vi "CAT Panel - MSR.vi"() -> ()   [LabVIEW 2012]
uses:
  <vilib>/Platform/TimedLoop/XDataNode/wakeup.ctl
  <vilib>/Platform/TimedLoop/XDataNode/XDNodeRunTimeDep.lvlib
  <vilib>/Platform/TimedLoop/XDataNode/nitl_modes.ctl
  <vilib>/Platform/TimedLoop/XDataNode/timing_clust.ctl
  <vilib>/Platform/TimedLoop/XDataNode/XDataNode.xnode
  Type Defs/Data Reading.ctl
  Type Defs/4 Way Button.ctl
  Output Timer/Output Timer.lvclass
  Type Defs/Alt Digit 100 New.ctl
  Type Defs/Alt Control.ctl
  Type Defs/All Timers.ctl
  Type Defs/Final Output for Dispaly.ctl
  Type Defs/Alt Display Large.ctl
  Type Defs/Final Output.ctl
  Type Defs/Output Values.ctl
  Type Defs/Output Switches.ctl
  Type Defs/CO2 Settings.ctl
  Type Defs/AD Settings.ctl
  Type Defs/Mode Select.ctl
  Type Defs/Action Time.ctl
  Type Defs/Timer Control.ctl
  Type Defs/Current Alt Set.ctl
  Altitude/Altitude.xctl
  Mode Control/Mode.xctl
panel:
  out "read string":string="Ver. 0.1, Feb 10 2013, 23:27:07\r\n"
  in  "Tab Control":T1(tab)=enum."CO2 Settings"
  in  "Other Outputs":cluster{"Alarm":bool, "Heater":bool}
  out "CO2 ppm":u32(slide)=831 scale=0.0..10000.0
  out "Alt Dif M":dbl(slide)=1598.2180776729308 scale=-1000.0..1000.0 scale format="%.1f"
  out "AD Output":T2
  out "AD State":T2
  out "Data Read":T3={"Date"="03/29/13", "Time"="15:49:08", "CO2- ppm"=831, "Last Ctrl Word"=4194304, "O2-1 ppm"=209373, "O2-2 ppm"=209370, "Temp MB"=21.72, "Temp Sensor Module"=23.23, "Press mB"=835.6} {"Last Ctrl Word" format="%.0x"}
  out "Force Output":T2
  out "Final Output":T2
  out "Force State":T2
  in  "CO2 Settings":T4={"Run C1"={"A-1,  1"=inf, "A-3,  2"=inf, "A-4, 3"=9000.0, "A-5, 4"=8800.0, "ABCD-7, 5"=9600.0, "A-8, 6"=9200.0, "B-1,  7"=3400.0, "B-3, 8"=3400.0, "B-4,  9"=9000.0, "B-5, 10"=8800.0, "B-8, 11"=9200.0, "C-1, 12"=1800.0, "C-3, 13"=1800.0, "C-4, 14"=9000.0, "C-5,  15"=8800.0, "C-8, 16"=9200.0, "D-1, 17"=inf, "D-3, 18"=3400.0, "D-4,  19"=1800.0, "D-5,  20"=7000.0, "D-8,  21"=9200.0}, "Run C2"={"A-1,  1"=inf, "A-3,  2"=inf, "A-4, 3"=8800.0, "A-5, 4"=8600.0, "ABCD-7, 5"=9400.0, "A-8, 6"=9000.0, "B-1,  7"=3000.0, "B-3, 8"=3000.0, "B-4,  9"=8800.0, "B-5, 10"=8600.0, "B-8, 11"=9000.0, "C-1, 12"=1400.0, "C-3, 13"=1400.0, "C-4, 14"=8800.0, "C-5,  15"=8600.0, "C-8, 16"=9000.0, "D-1, 17"=inf, "D-3, 18"=3000.0, "D-4,  19"=1400.0, "D-5,  20"=6600.0, "D-8,  21"=9000.0}, "Hold C3"={"A-1,  1"=1800.0, "A-3,  2"=1800.0, "A-4, 3"=9000.0, "A-5, 4"=8800.0, "ABCD-7, 5"=9600.0, "A-8, 6"=9200.0, "B-1,  7"=3400.0, "B-3, 8"=3400.0, "B-4,  9"=9000.0, "B-5, 10"=8800.0, "B-8, 11"=9200.0, "C-1, 12"=1800.0, "C-3, 13"=1800.0, "C-4, 14"=9000.0, "C-5,  15"=8800.0, "C-8, 16"=9200.0, "D-1, 17"=1800.0, "D-3, 18"=3400.0, "D-4,  19"=1800.0, "D-5,  20"=7000.0, "D-8,  21"=9200.0}, "Hold C4"={"A-1,  1"=1400.0, "A-3,  2"=1400.0, "A-4, 3"=8800.0, "A-5, 4"=8600.0, "ABCD-7, 5"=9400.0, "A-8, 6"=9000.0, "B-1,  7"=3000.0, "B-3, 8"=3000.0, "B-4,  9"=8800.0, "B-5, 10"=8600.0, "B-8, 11"=9000.0, "C-1, 12"=1400.0, "C-3, 13"=1400.0, "C-4, 14"=8800.0, "C-5,  15"=8600.0, "C-8, 16"=9000.0, "D-1, 17"=1400.0, "D-3, 18"=3000.0, "D-4,  19"=1400.0, "D-5,  20"=6600.0, "D-8,  21"=9000.0}, "High CO2 Forces "={"A-1, 1"=TRUE, "A-3, 2"=TRUE, "A-4, 3"=FALSE, "A-5, 4"=TRUE, "ABCD-7, 5"=FALSE, "A-8, 6"=TRUE, "B-1,  7"=TRUE, "B-3, 8"=TRUE, "B-4, 9"=FALSE, "B-5, 10"=TRUE, "B-8,  11"=TRUE, "C-1, 12"=TRUE, "C-3, 13"=TRUE, "C-4,  14"=FALSE, "C-5,  15"=TRUE, "C-8, 16"=TRUE, "D-1, 17"=TRUE, "D-3, 18"=TRUE, "D-4, 19"=TRUE, "D-5,  20"=TRUE, "D-8,  21"=TRUE}}
  in  "AD Settings":T7={"Set Point Force"={"A-1,  1"=inf, "A-3,  2"=inf, "A-4, 3"=inf, "A-5, 4"=inf, "ABCD-7, 5"=inf, "A-8, 6"=inf, "B-1,  7"=inf, "B-3, 8"=inf, "B-4,  9"=inf, "B-5, 10"=inf, "B-8, 11"=inf, "C-1, 12"=inf, "C-3, 13"=inf, "C-4, 14"=inf, "C-5,  15"=inf, "C-8, 16"=inf, "D-1, 17"=inf, "D-3, 18"=inf, "D-4,  19"=inf, "D-5,  20"=6000.0, "D-8,  21"=inf}, "Run A1"={"A-1,  1"=inf, "A-3,  2"=inf, "A-4, 3"=50.0, "A-5, 4"=inf, "ABCD-7, 5"=150.0, "A-8, 6"=60.0, "B-1,  7"=0.0, "B-3, 8"=0.0, "B-4,  9"=50.0, "B-5, 10"=inf, "B-8, 11"=60.0, "C-1, 12"=15.0, "C-3, 13"=15.0, "C-4, 14"=50.0, "C-5,  15"=inf, "C-8, 16"=60.0, "D-1, 17"=inf, "D-3, 18"=0.0, "D-4,  19"=15.0, "D-5,  20"=0.0, "D-8,  21"=700.0}, "Run A2"={"A-1,  1"=inf, "A-3,  2"=inf, "A-4, 3"=-30.0, "A-5, 4"=inf, "ABCD-7, 5"=80.0, "A-8, 6"=15.0, "B-1,  7"=-80.0, "B-3, 8"=-80.0, "B-4,  9"=-30.0, "B-5, 10"=inf, "B-8, 11"=15.0, "C-1, 12"=-50.0, "C-3, 13"=-50.0, "C-4, 14"=-30.0, "C-5,  15"=inf, "C-8, 16"=15.0, "D-1, 17"=inf, "D-3, 18"=0.0, "D-4,  19"=-50.0, "D-5,  20"=-80.0, "D-8,  21"=650.0}, "Hold A3"={"A-1,  1"=0.0, "A-3,  2"=0.0, "A-4, 3"=50.0, "A-5, 4"=inf, "ABCD-7, 5"=150.0, "A-8, 6"=60.0, "B-1,  7"=-150.0, "B-3, 8"=-150.0, "B-4,  9"=50.0, "B-5, 10"=inf, "B-8, 11"=60.0, "C-1, 12"=-200.0, "C-3, 13"=-200.0, "C-4, 14"=50.0, "C-5,  15"=inf, "C-8, 16"=60.0, "D-1, 17"=0.0, "D-3, 18"=-150.0, "D-4,  19"=-200.0, "D-5,  20"=-200.0, "D-8,  21"=650.0}, "Hold A4"={"A-1,  1"=-150.0, "A-3,  2"=-150.0, "A-4, 3"=-30.0, "A-5, 4"=inf, "ABCD-7, 5"=80.0, "A-8, 6"=15.0, "B-1,  7"=-250.0, "B-3, 8"=-250.0, "B-4,  9"=-30.0, "B-5, 10"=inf, "B-8, 11"=15.0, "C-1, 12"=-300.0, "C-3, 13"=-300.0, "C-4, 14"=-30.0, "C-5,  15"=inf, "C-8, 16"=15.0, "D-1, 17"=-150.0, "D-3, 18"=-250.0, "D-4,  19"=-300.0, "D-5,  20"=-300.0, "D-8,  21"=650.0}, "High AD Diff "={"A-1, 1"=FALSE, "A-3, 2"=FALSE, "A-4, 3"=FALSE, "A-5, 4"=TRUE, "ABCD-7, 5"=FALSE, "A-8, 6"=TRUE, "B-1,  7"=FALSE, "B-3, 8"=FALSE, "B-4, 9"=FALSE, "B-5, 10"=TRUE, "B-8,  11"=TRUE, "C-1, 12"=FALSE, "C-3, 13"=FALSE, "C-4,  14"=FALSE, "C-5,  15"=TRUE, "C-8, 16"=TRUE, "D-1, 17"=FALSE, "D-3, 18"=FALSE, "D-4, 19"=FALSE, "D-5,  20"=FALSE, "D-8,  21"=TRUE}, "Delay S"={"A-1,  1"=30.0, "A-3,  2"=30.0, "A-4, 3"=1.0, "A-5, 4"=1.0, "ABCD-7, 5"=1.0, "A-8, 6"=1.0, "B-1,  7"=30.0, "B-3, 8"=30.0, "B-4,  9"=1.0, "B-5, 10"=1.0, "B-8, 11"=1.0, "C-1, 12"=30.0, "C-3, 13"=30.0, "C-4, 14"=1.0, "C-5,  15"=1.0, "C-8, 16"=1.0, "D-1, 17"=30.0, "D-3, 18"=30.0, "D-4,  19"=30.0, "D-5,  20"=30.0, "D-8,  21"=1.0}}
  in  "Main States":T8(tab)=enum."Setup"
  out "ALT DISPLAY":sgl format="%#.0f"
  out "CURRENT ALT SET":T9=1598 format="%#.0f"
  in  "Mode 1":T10
  in  "Confirm Now 2":bool
  out "Carbon Dioxide  %":sgl=0.0831 format="%.3f"
  in  "ALT SET 2":T11 {"Alt Digit 100" min=0 max=9 step=1; "Alt Digit 100" min=0 max=9 step=1; "Alt Digit 100" min=0 max=9 step=1; "Alt Digit 100" min=0 max=9 step=1; "Alt Digit 100" min=0 max=9 step=1}
  out "ALT DISPLAY 2":T13=1598.218 format="%#.0f"
  out "CURRENT ALT SET 2":T9=1598 format="%#.0f"
  in  "Mode":T10
  out "Time":string="15:49:02"
  in  "Add Note":bool
  out "Final Output Display":T14
  out "CO2 Chart":dbl(graph)=0.0831
  out "Temp C":sgl=21.69
  out "Press mB":sgl=835.53
  out "Date":string="03/29/13"
  out "Alt Chart":dbl(graph)=1598.2180776729308
  out "Carbon Dioxide":sgl=0.0831 format="%.3g"
  in  "Confirm Now":bool
  in  "Notes":string
  in  "ALT SET":T11 {"Alt Digit 100" min=0 max=9 step=1; "Alt Digit 100" min=0 max=9 step=1; "Alt Digit 100" min=0 max=9 step=1; "Alt Digit 100" min=0 max=9 step=1; "Alt Digit 100" min=0 max=9 step=1}
  out "Altitude":sgl=1598.218 format="%#.0f"
  out "O2%":dbl=21.4333 format="%.1f"
  in  "Timers":T15 {"Timer 4"."Action Time" format="%<%H:%M>t"; "Timer 3"."Action Time" format="%<%H:%M>t"; "Timer 2"."Action Time" format="%<%H:%M>t"; "Timer"."Action Time" format="%<%H:%M>t"}
  in  "Datalog File":path
  in  "Period mS":i64=6000
  in  "Stop Button":bool
  in  "West ON/Std OFF":bool
  out "error out":errorcluster
  out "Cycles":i32=5
  in  "Mode Select":T18
  in  "Set Point Alt":sgl min=0 max=10000 step=1
  # "CAT 100.8"
  # "Current Effective Altitude in  Meters"
  # "M\nE\nT\nE\nR\nS"
  # "%"
  # "Channel A"
  # "Channel B"
  # "Channel C"
  # "Channel D"
  # "1"
  # "1"
  # "1"
  # "1"
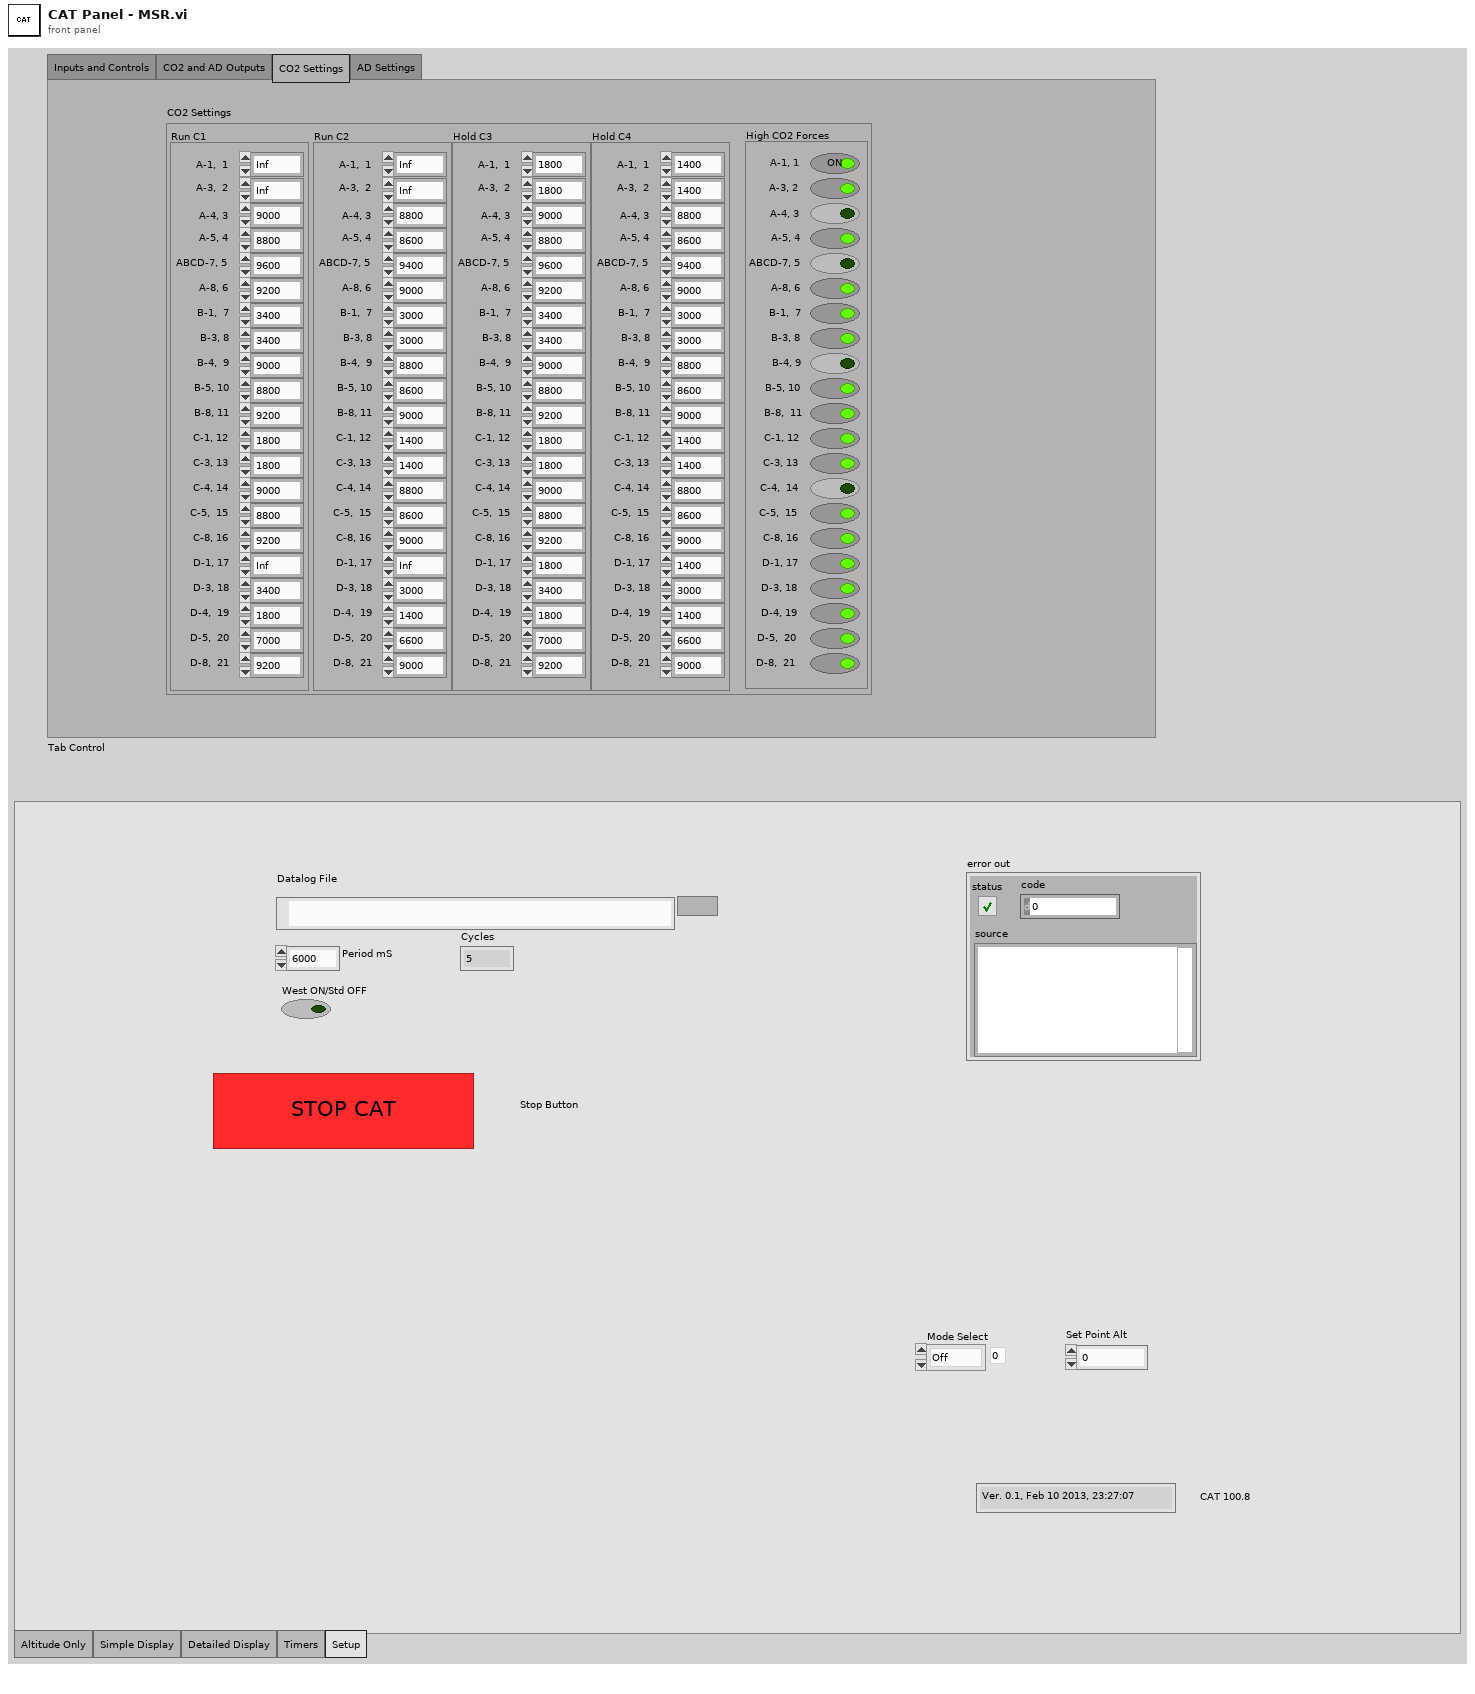
[diagram p1: front panel]
types:
  T1 = enum32{"Inputs and Controls", "CO2 and AD Outputs", "CO2 Settings", "AD Settings"}
  T2 = typedef "Final Output.ctl" = cluster{"Main 1":bool, "Main 2":bool, "Recirc  3":bool, "Scrub 4":bool, "O2 5":bool, "Vent 6":bool, "Boost A 7":bool, "Boost A 8":bool, "Recirc  9":bool, "Scrub 10":bool, "Vent 11":bool, "Boost B 12":bool, "Boost B 13":bool, "Recirc 14":bool, "Scrub 15":bool, "Vent 16":bool, "Main 17":bool, "Boost A 18":bool, "Boost B 19":bool, "Boost F 20":bool, "Vent 2 21":bool}
  T3 = typedef "Data Reading.ctl" = cluster{"Date":string, "Time":string, "CO2- ppm":u32, "Last Ctrl Word":u32, "O2-1 ppm":u32, "O2-2 ppm":u32, "Temp MB":sgl, "Temp Sensor Module":sgl, "Press mB":sgl}
  T4 = typedef "CO2 Settings.ctl" = cluster{"Run C1":T5, "Run C2":T5, "Hold C3":T5, "Hold C4":T5, "High CO2 Forces ":T6}
  T5 = typedef "Output Values.ctl" = cluster{"A-1,  1":dbl, "A-3,  2":dbl, "A-4, 3":dbl, "A-5, 4":dbl, "ABCD-7, 5":dbl, "A-8, 6":dbl, "B-1,  7":dbl, "B-3, 8":dbl, "B-4,  9":dbl, "B-5, 10":dbl, "B-8, 11":dbl, "C-1, 12":dbl, "C-3, 13":dbl, "C-4, 14":dbl, "C-5,  15":dbl, "C-8, 16":dbl, "D-1, 17":dbl, "D-3, 18":dbl, "D-4,  19":dbl, "D-5,  20":dbl, "D-8,  21":dbl}
  T6 = typedef "Output Switches.ctl" = cluster{"A-1, 1":bool, "A-3, 2":bool, "A-4, 3":bool, "A-5, 4":bool, "ABCD-7, 5":bool, "A-8, 6":bool, "B-1,  7":bool, "B-3, 8":bool, "B-4, 9":bool, "B-5, 10":bool, "B-8,  11":bool, "C-1, 12":bool, "C-3, 13":bool, "C-4,  14":bool, "C-5,  15":bool, "C-8, 16":bool, "D-1, 17":bool, "D-3, 18":bool, "D-4, 19":bool, "D-5,  20":bool, "D-8,  21":bool}
  T7 = typedef "AD Settings.ctl" = cluster{"Set Point Force":T5, "Run A1":T5, "Run A2":T5, "Hold A3":T5, "Hold A4":T5, "High AD Diff ":T6, "Delay S":T5}
  T8 = enum32{"Altitude Only", "Simple Display", "Detailed Display", "Timers", "Setup"}
  T9 = typedef "Current Alt Set.ctl" = i32
  T10 = typedef "4 Way Button.ctl" = cluster{"Off":bool, "Standby":bool, "Hold":bool, "Run":bool}
  T11 = typedef "Alt Control.ctl" = cluster{"Alt Digit 100":T12, "Alt Digit 100":T12, "Alt Digit 100":T12, "Alt Digit 100":T12, "Alt Digit 100":T12}
  T12 = typedef "Alt Digit 100 New.ctl" = i8
  T13 = typedef "Alt Display Large.ctl" = sgl
  T14 = typedef "Final Output for Dispaly.ctl" = cluster{"A-1,  1":bool, "A-3,  2":bool, "A-4, 3":bool, "A-5, 4":bool, "ABCD-7, 5":bool, "A-8, 6":bool, "B-1,  7":bool, "B-3, 8":bool, "B-4,  9":bool, "B-5, 10":bool, "B-8, 11":bool, "C-1, 12":bool, "C-3, 13":bool, "C-4, 14":bool, "C-5,  15":bool, "C-8, 16":bool, "A-1, 17":bool, "D-3, 18":bool, "D-4,  19":bool, "D-5,  20":bool, "D-8,  21":bool}
  T15 = typedef "All Timers.ctl" = cluster{"Timer":T16, "Timer 2":T16, "Timer 3":T16, "Timer 4":T16}
  T16 = typedef "Timer Control.ctl" = cluster{"Sun":bool, "Timer":bool, "Altitude":sgl, "Action Time":T17, "Mon":bool, "Tues":bool, "Wed":bool, "Thur":bool, "Fri":bool, "Sat":bool, "Mode":enum8{"Off", "Stby", "Hold", "Run"}}
  T17 = typedef "Action Time.ctl" = dbl
  T18 = typedef "Mode Select.ctl" = enum8{"Off", "Stby", "Hold", "Run"}
  T19 = cluster{"Main 1":bool, "Main 2":bool, "Recirc  3":bool, "Boost A 7":bool, "Recirc  9":bool, "Scrub 4":bool, "Scrub 10":bool, "O2 5":bool, "Vent 6":bool, "Boost A 8":bool, "Vent 11":bool, "Boost B 12":bool, "Boost B 13":bool, "Recirc 14":bool, "Scrub 15":bool, "Vent 16":bool, "Main 17":bool, "Boost A 18":bool, "Boost B 19":bool, "Boost F 20":bool, "Vent 2 21":bool}
  T20 = typedef "XDNodeRunTimeDep.lvlib/timing_clust.ctl" = cluster{"Expected End [f-1]":u64, "Actual End [f-1]":u64, "Finished Late? [f-1]":bool, "Expected End [i-1]":u64, "Actual End [i-1]":u64, "Finished Late? [i-1]":bool, "Expected Start [i]":u64, "Actual Start [i]":u64, "Expected Start [f]":u64, "Actual Start [f]":u64, "Source Name":string, "Structure Name":string, "Period":i64, "Deadline":i64, "Offset":i64, "Start":i64, "Priority":i32, "Timeout":i32, "Mode":T21, "Wakeup Reason":T22, "Error":errorcluster, "Source Type":string, "Secondary Source Type":string, "Global End Time":u64, "Global Start Time":u64, "Frame Duration":u64, "Iteration Duration":u64, "Assigned CPU":i32, "I/O Scan Engine Mode":u32}
  T21 = typedef "XDNodeRunTimeDep.lvlib/nitl_modes.ctl" = enum32{"No Change", "Process missed periods, maintain original phase", "Discard missed periods, maintain original phase", "Process missed periods, ignore original phase", "Discard missed periods, ignore original phase"}
  T22 = typedef "XDNodeRunTimeDep.lvlib/wakeup.ctl" = enum32{"Normal", "Aborted", "Asynchronous wakeup", "Timing source error", "Timed loop error", "Timeout"}
  T23 = cluster{"A-1,  1":bool, "A-3,  2":bool, "A-4, 3":bool, "A-5, 4":bool, "ABCD-7, 5":bool, "A-8, 6":bool, "B-1,  7":bool, "B-3, 8":bool, "B-4,  9":bool, "B-5, 10":bool, "B-8, 11":bool, "C-1, 12":bool, "C-3, 13":bool, "C-4, 14":bool, "C-5,  15":bool, "C-8, 16":bool, "D-1, 17":bool, "D-3, 18":bool, "D-4,  19":bool, "D-5,  20":bool, "D-8,  21":bool}
  T24 = cluster{bool, bool, bool, bool, bool, bool, bool, bool, bool, bool, bool, bool, bool, bool, bool, bool, bool, bool, bool, bool, bool}
  T25 = cluster{"[0]":bool, "[1]":bool, "[2]":bool, "[3]":bool, "[4]":bool, "[5]":bool, "[6]":bool, "[7]":bool, "[8]":bool, "[9]":bool, "[10]":bool, "[11]":bool, "[12]":bool, "[13]":bool, "[14]":bool, "[15]":bool, "[16]":bool, "[17]":bool, "[18]":bool, "[19]":bool, "[20]":bool}
  T26 = cluster{"Date":string, "Time":string, "CO2- ppm":u32, "Last Ctrl Word":u32, "O2-1 ppm":u32, "O2-2 ppm":u32, "Temp MB":sgl, "Temp Sensor Module":sgl, "Press mB":sgl}
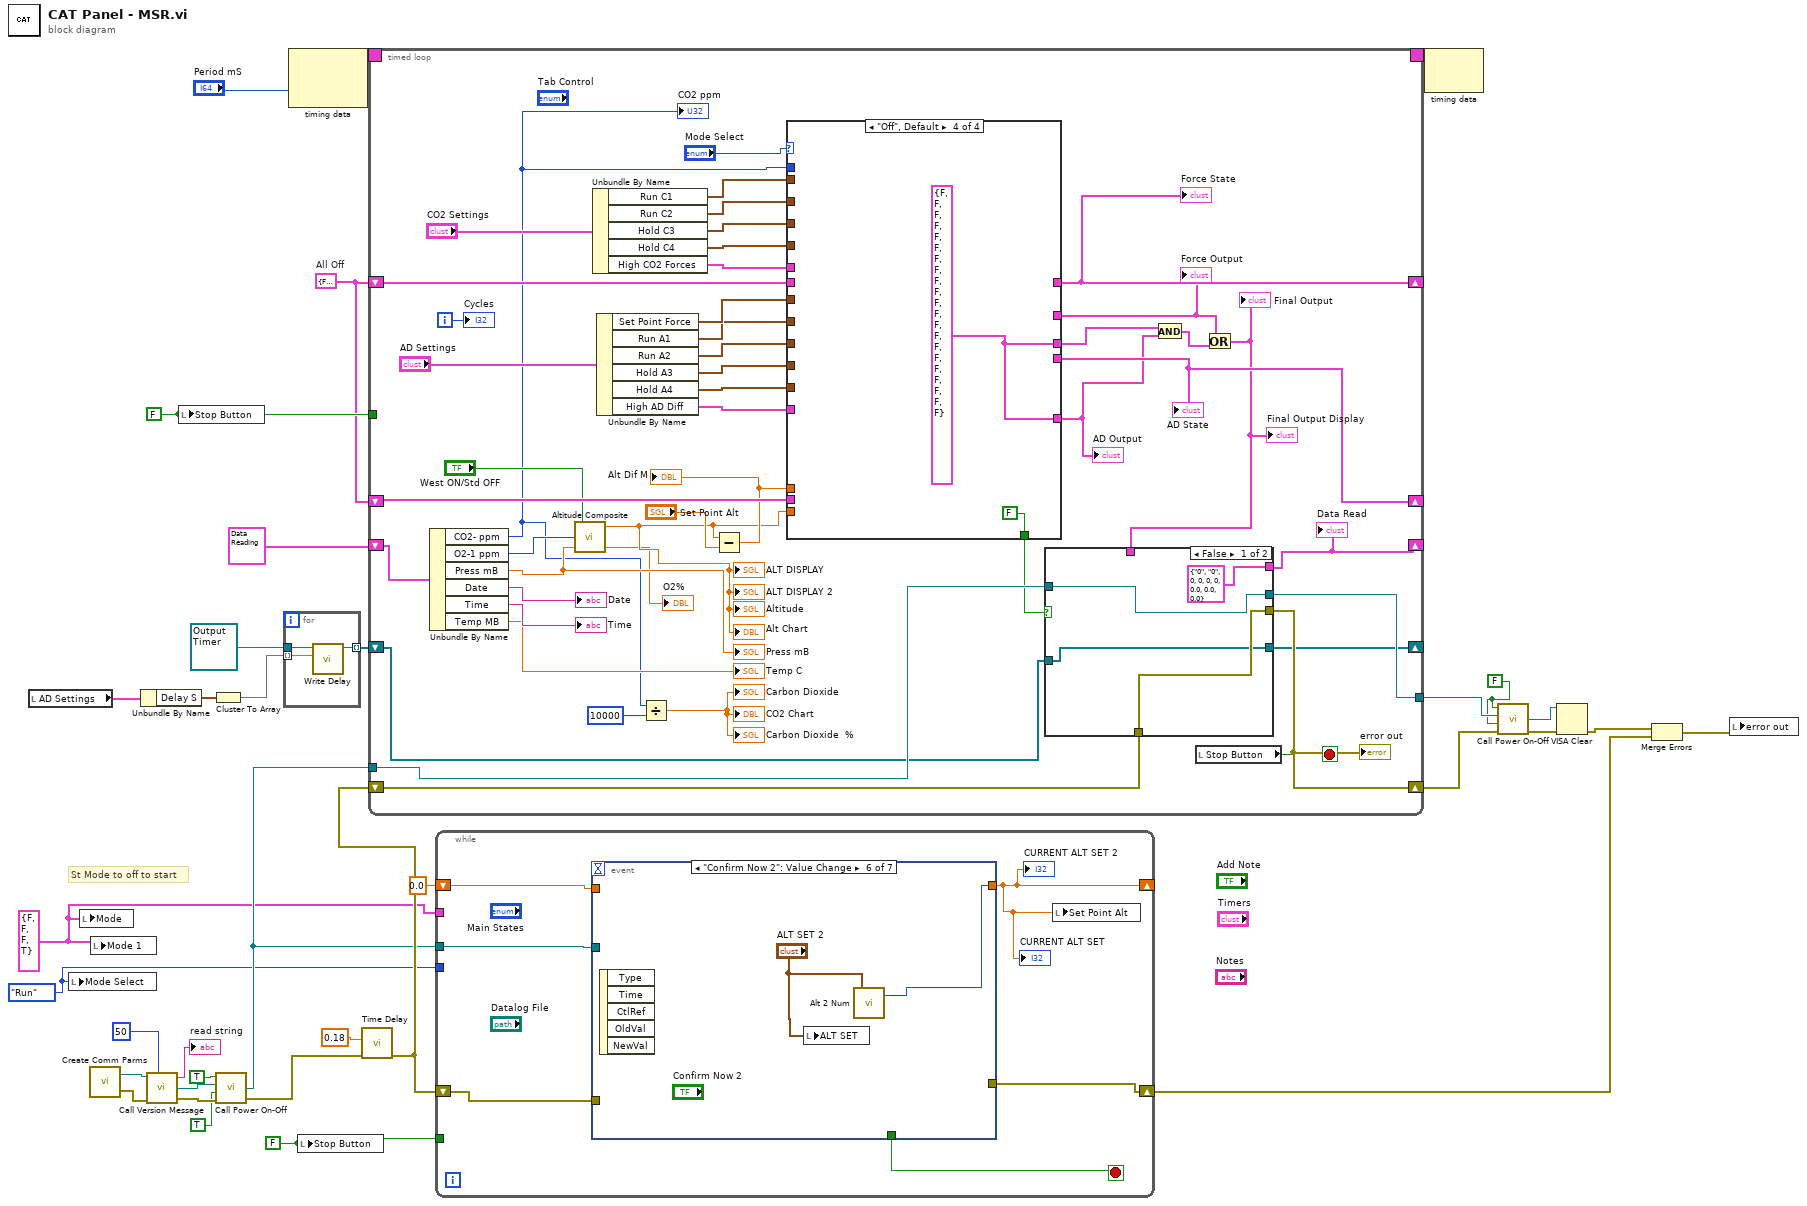
[diagram p0: block diagram]
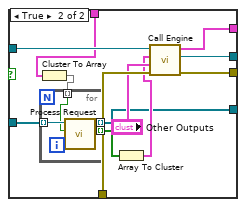
[diagram p2: hidden frame]
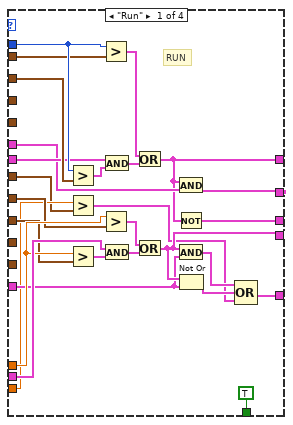
[diagram p3: hidden frame]
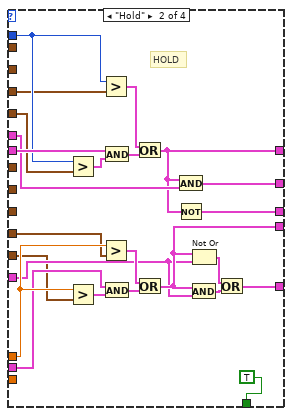
[diagram p4: hidden frame]
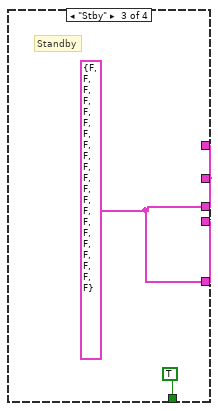
[diagram p5: hidden frame]
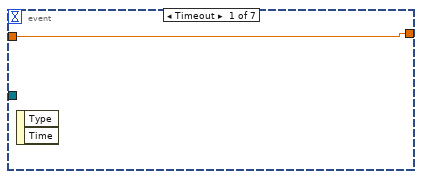
[diagram p6: hidden frame]
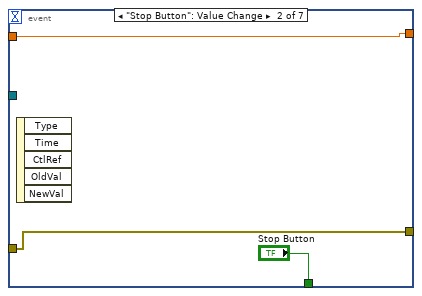
[diagram p7: hidden frame]
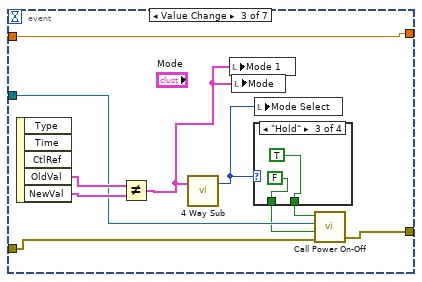
[diagram p8: hidden frame]
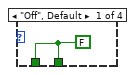
[diagram p9: hidden frame]
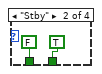
[diagram p10: hidden frame]
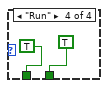
[diagram p11: hidden frame]
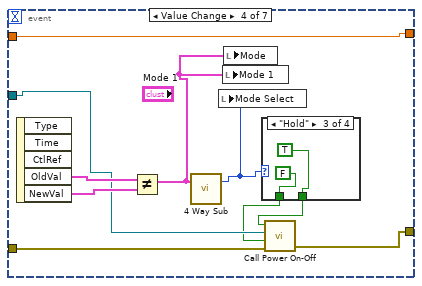
[diagram p12: hidden frame]
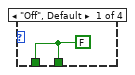
[diagram p13: hidden frame]
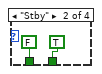
[diagram p14: hidden frame]
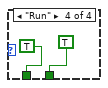
[diagram p15: hidden frame]
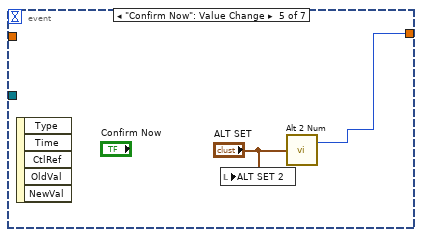
[diagram p16: hidden frame]
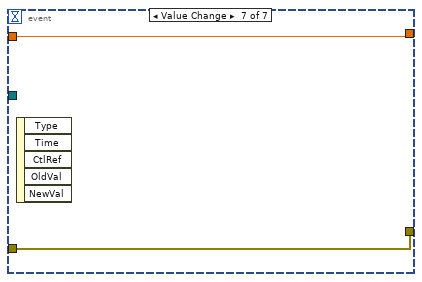
[diagram p17: hidden frame]
diagram:
  w1 = FALSE ("Leave CAT On/Off at Program Exit")
  w12 = T10 {"Off"=FALSE, "Standby"=FALSE, "Hold"=FALSE, "Run"=TRUE} ("Mode 1")
  w13 = enum8{"Off", "Stby", "Hold", "Run"}."Run" ("Mode Select")
  w31 = FALSE ("Stop Button")
  w32 = FALSE ("Stop Button")
  w30 = T19 {"Main 1"=FALSE, "Main 2"=FALSE, "Recirc  3"=FALSE, "Boost A 7"=FALSE, "Recirc  9"=FALSE, "Scrub 4"=FALSE, "Scrub 10"=FALSE, "O2 5"=FALSE, "Vent 6"=FALSE, "Boost A 8"=FALSE, "Vent 11"=FALSE, "Boost B 12"=FALSE, "Boost B 13"=FALSE, "Recirc 14"=FALSE, "Scrub 15"=FALSE, "Vent 16"=FALSE, "Main 17"=FALSE, "Boost A 18"=FALSE, "Boost B 19"=FALSE, "Boost F 20"=FALSE, "Vent 2 21"=FALSE}  # All Off
  # "St Mode to off to start"
  n1 = local read "AD Settings"() -> (w11:T7)
  n2 = local write "Mode Select"(w13) -> ()
  n3 = local write "Mode"(w12) -> ()
  n4 = call "Create Comm Parms.vi"() -> ("error out"=w19:errorcluster, "VISA resource name out"=w17:refnum<visa-resource-name>)  [unwired: 2 in]
  n5 = local write "Mode 1"(w12) -> ()
  n6 = Unbundle By Name(w11) -> ("Delay S"=w10:T5)
  n7 = call "Call Version Message.vi"("VISA resource name out"=w17, "delay before read (ms)"=u32 50, "error in"=w19) -> ("read string"=→"read string":string, "VISA resource name out 2"=w16:refnum<visa-resource-name>, "error out"=w18:errorcluster)  [unwired: 2 in, 1 out]
  n8 = local write "Stop Button"(w32) -> ()
  n9 = Cluster To Array(cluster=w10) -> (array=w9:dbl[])
  n10 = call "Call Power On-Off.vi"("error in"=w18, "Warmup if ON"=TRUE, "VISA resource name"=w16, "On/Off"=TRUE) -> ("error out"=w28:errorcluster, "VISA resource name out"=w22:refnum<visa-resource-name>)  [unwired: 1 in]
  n11 = for {
    tunnel: w9 -> [w37] mode=indexing
    tunnel: refnum<class "Output Timer.lvclass"> refnum ("Delay Timer") -> [w38]
    tunnel: [w36] -> w7 mode=indexing
    n12 = call "Write Delay.vi"("Delay"=w37, "Output Timer in"=w38) -> ("Output Timer out"=w36:refnum<class "Output Timer.lvclass">)  [unwired: 8 in, 1 out]
  }
  n13 = node-c288("Period mS") -> (w35:T20)  [unwired: 1 in]
  n14 = local write "Stop Button"(w31) -> ()
  n15 = call "Time Delay"("error in (no error)"=w28, "Delay Time (s)"=0.18) -> ("error out"=w23:errorcluster)  [unwired: 9 in]
  n16 = timed-loop {
    shift-right: [w85] -> _
    shift-left: w30 -> [w84]
    shift-right: [w82] -> _
    shift-left: w30 -> [w81]
    timing: w35 -> [_]
    timing-out: [_] -> w34
    shift-right: [w62] -> w24
    shift-left: w23 -> [w63]
    shift-right: [w61] -> _
    shift-left: T3 {"Date"="", "Time"="", "CO2- ppm"=380, "Last Ctrl Word"=0, "O2-1 ppm"=209400, "O2-2 ppm"=209400, "Temp MB"=20.0, "Temp Sensor Module"=20.0, "Press mB"=1013.0} ("Data Read") -> [w60]
    tunnel: w32 -> [_]
    tunnel: [w45] -> w20
    tunnel: w22 -> [w46]
    shift-right: [w40] -> _
    shift-left: w7 -> [w41]
    i -> [w83]
    stop <- w47 stop-if-true
    n17 = Unbundle By Name(w60) -> ("CO2- ppm"=w52:u32, "O2-1 ppm"=w58:u32, "Press mB"=w53:sgl, "Date"=→"Date":string, "Time"=→"Time":string, "Temp MB"=→"Temp C":sgl)
    "CO2 ppm" <- w52
    "Press mB" <- w53
    n18 = call "Altitude Composite.vi"("Pressure mBar"=w53, "O2ppm"=w58, "West ON/Std OFF"="West ON/Std OFF") -> ("O2%"=→"O2%":dbl, "Alt Eff M 1 correct"=w48:dbl)  [unwired: 1 out]
    "ALT DISPLAY" <- w48
    "Altitude" <- w48
    "ALT DISPLAY 2" <- w48
    "Alt Chart" <- w48
    n19 = Unbundle By Name("CO2 Settings") -> ("Run C1"=w64:T5, "Run C2"=w65:T5, "Hold C3"=w66:T5, "Hold C4"=w67:T5, "High CO2 Forces"=w68:T6)
    n20 = Unbundle By Name("AD Settings") -> ("Set Point Force"=w75:T5, "Run A1"=w74:T5, "Run A2"=w73:T5, "Hold A3"=w72:T5, "Hold A4"=w71:T5, "High AD Diff"=w70:T6)
    n21 = Divide(x=w52, y=u32 10000) -> (x/y=→"Carbon Dioxide" →"Carbon Dioxide  %" →"CO2 Chart":dbl)
    n22 = Subtract(x=w48, y="Set Point Alt") -> (x-y=w57:dbl)
    "Alt Dif M" <- w57
    n23 = case shown="\"Off\", Default" "Mode Select" {
      tunnel: w52 -> [w131 w153 _ _]
      tunnel: w64 -> [w130 _ _ _]
      tunnel: [w108 w137 w158 _] -> w85
      tunnel: w65 -> [w132 _ _ _]
      tunnel: w66 -> [_ w152 _ _]
      tunnel: w67 -> [_ w151 _ _]
      tunnel: w84 -> [w127 w154 _ _]
      tunnel: w68 -> [w109 w143 _ _]
      tunnel: [w118 w144 w158 _] -> w80
      tunnel: w57 -> [w123 w148 _ _]
      tunnel: w74 -> [w122 _ _ _]
      tunnel: w73 -> [w121 _ _ _]
      tunnel: w72 -> [_ w135 _ _]
      tunnel: w71 -> [_ w134 _ _]
      tunnel: w70 -> [w116 w141 _ _]
      tunnel: [w117 w142 w158 _] -> w82
      tunnel: w81 -> [w124 w147 _ _]
      tunnel: [w110 w138 w158 w160] -> w79
      tunnel: w48 -> [w113 _ _ _]
      tunnel: w75 -> [w112 _ _ _]
      tunnel: [w107 w136 w158 w160] -> w78
      tunnel: [TRUE TRUE TRUE FALSE] -> w43
      frame "Run" {
        # "RUN"
        n24 = Greater?(x=w131, y=w132) -> (0:w120:T23)
        n25 = Greater?(x=w113, y=w112) -> (0:w111:T23)
        n26 = Greater?(x=w123, y=w121) -> (0:w119:T23)
        n27 = Greater?(x=w131, y=w130) -> (0:w129:T23)
        n28 = Greater?(x=w123, y=w122) -> (0:w126:T23)
        n29 = And(x=w127, y=w120) -> (x .and. y?=w128:T24)
        n30 = And(x=w124, y=w119) -> (x .and. y?=w125:T24)
        n31 = Or(x=w129, y=w128) -> (x .or. y?=w108:T24)
        n32 = Or(x=w126, y=w125) -> (x .or. y?=w117:T24)
        n33 = And(x=w108, y=w109) -> (x .and. y?=w118:T6)
        n34 = Not(x=w108) -> (.not. x?=w107:T24)
        n35 = And(x=w117, y=w116) -> (x .and. y?=w115:T6)
        n36 = Not Or(1:w116, 2:w117) -> (0:w114:T6)
        n37 = Compound Arithmetic op=OR(w115, w114, w111) -> (w110:T6)
      }
      frame "Hold" {
        # "HOLD"
        n38 = Greater?(x=w153, y=w151) -> (0:w146:T23)
        n39 = Greater?(x=w148, y=w134) -> (0:w145:T23)
        n40 = Greater?(x=w153, y=w152) -> (0:w156:T23)
        n41 = Greater?(x=w148, y=w135) -> (0:w150:T23)
        n42 = And(x=w154, y=w146) -> (x .and. y?=w155:T24)
        n43 = And(x=w147, y=w145) -> (x .and. y?=w149:T24)
        n44 = Or(x=w156, y=w155) -> (x .or. y?=w137:T24)
        n45 = Or(x=w150, y=w149) -> (x .or. y?=w142:T24)
        n46 = And(x=w137, y=w143) -> (x .and. y?=w144:T6)
        n47 = Not(x=w137) -> (.not. x?=w136:T24)
        n48 = Not Or(1:w141, 2:w142) -> (0:w140:T6)
        n49 = And(x=w142, y=w141) -> (x .and. y?=w139:T6)
        n50 = Or(x=w140, y=w139) -> (x .or. y?=w138:T6)
      }
      frame "Stby" {
        w158 = T19 {"Main 1"=FALSE, "Main 2"=FALSE, "Recirc  3"=FALSE, "Boost A 7"=FALSE, "Recirc  9"=FALSE, "Scrub 4"=FALSE, "Scrub 10"=FALSE, "O2 5"=FALSE, "Vent 6"=FALSE, "Boost A 8"=FALSE, "Vent 11"=FALSE, "Boost B 12"=FALSE, "Boost B 13"=FALSE, "Recirc 14"=FALSE, "Scrub 15"=FALSE, "Vent 16"=FALSE, "Main 17"=FALSE, "Boost A 18"=FALSE, "Boost B 19"=FALSE, "Boost F 20"=FALSE, "Vent 2 21"=FALSE}
        # "Standby"
      }
      frame "Off", Default {
        w160 = T19 {"Main 1"=FALSE, "Main 2"=FALSE, "Recirc  3"=FALSE, "Boost A 7"=FALSE, "Recirc  9"=FALSE, "Scrub 4"=FALSE, "Scrub 10"=FALSE, "O2 5"=FALSE, "Vent 6"=FALSE, "Boost A 8"=FALSE, "Vent 11"=FALSE, "Boost B 12"=FALSE, "Boost B 13"=FALSE, "Recirc 14"=FALSE, "Scrub 15"=FALSE, "Vent 16"=FALSE, "Main 17"=FALSE, "Boost A 18"=FALSE, "Boost B 19"=FALSE, "Boost F 20"=FALSE, "Vent 2 21"=FALSE}
      }
    }
    "Force State" <- w85
    "Force Output" <- w80
    "AD State" <- w82
    "AD Output" <- w79
    n51 = And(x=w78, y=w79) -> (x .and. y?=w77:T6)
    n52 = local read "Stop Button"() -> (w47:bool)
    n53 = Or(x=w80, y=w77) -> (x .or. y?=w44:T6)
    "Final Output" <- w44
    "Final Output Display" <- w44
    n54 = case shown="False" w43 {
      tunnel: w63 -> [w89 w101]
      tunnel: [w89 w100] -> w62
      tunnel: [T3 {"Date"="0", "Time"="0", "CO2- ppm"=0, "Last Ctrl Word"=0, "O2-1 ppm"=0, "O2-2 ppm"=0, "Temp MB"=0.0, "Temp Sensor Module"=0.0, "Press mB"=0.0} ("Data Read") w99] -> w61
      tunnel: w46 -> [w87 w97]
      tunnel: [w87 w96] -> w45
      tunnel: w44 -> [_ w95]
      tunnel: w41 -> [w86 w94]
      tunnel: [w86 w90] -> w40
      frame False {
      }
      frame True {
        n55 = Cluster To Array(cluster=w95) -> (array=w93:bool[])
        n56 = for {
          tunnel: w94 -> [w105] mode=indexing
          tunnel: w93 -> [w104] mode=indexing
          tunnel: [w103] -> w90 mode=indexing
          tunnel: [w102] -> w92 mode=indexing
          n57 = call "Process Request.vi"("Requested"=w104, "Delay Timer in"=w105) -> ("Returned"=w102:bool, "Delay Timer out"=w103:refnum<class "Output Timer.lvclass">)  [unwired: 7 in, 1 out]
        }
        n58 = Array To Cluster(array=w92) -> (cluster=w91:T25)
        n59 = call "Call Engine.vi"("error in"=w101, "Other Outputs"="Other Outputs", "Final Output Controls"=w91, "Port"=w97) -> ("error out"=w100:errorcluster, "VISA resource name out"=w96:refnum<visa-resource-name>, "Data Read"=w99:T26)  [unwired: 1 in, 1 out]
      }
    }
    "error out" <- w62
    "Data Read" <- w61
    "Cycles" <- w83
  }
  n60 = while {
    tunnel: w31 -> [_]
    shift-right: [w166] -> w26
    shift-left: w23 -> [w167]
    tunnel: w22 -> [w165]
    tunnel: w13 -> [_]
    tunnel: w12 -> [_]
    shift-right: [w163] -> _
    shift-left: sgl 0.0 ("Alt") -> [w164]
    stop <- w168 stop-if-true
    n61 = event shown="[5] \"Confirm Now 2\": Value Change" {
      selector: _ -> [_ _ _ _ _ _ _]
      dyn-events: _ -> [_ _ _ _ _ _ _]
      timeout: _ -> [_ _ _ _ _ _ _]
      tunnel: [w169 w170 w174 w193 w208 w210 w212] -> w163
      tunnel: [_ "Stop Button" _ _ _ _ _] -> w168
      tunnel: w167 -> [_ w171 w179 w196 _ _ w211]
      tunnel: [_ w171 w178 w195 _ _ w211] -> w166
      tunnel: w165 -> [_ _ w177 w194 _ _ _]
      tunnel: w164 -> [w169 w170 w174 w193 _ _ w212]
      event Timeout {
        n62 = event-data() -> ()  [unwired: 1 in, 2 out]
      }
      event "Stop Button": Value Change {
        n63 = event-data() -> ()  [unwired: 1 in, 5 out]
      }
      event Value Change {
        n64 = event-data() -> ("OldVal"=w182:T10, "NewVal"=w181:T10)  [unwired: 1 in, 3 out]
        n65 = Not Equal?(x=w182, y=w181) -> (x != y?=w180:T10)
        n66 = call "4 Way Sub.vi"("OldVal"=w180) -> ("Mode Select"=w175:enum8{"Off", "Stby", "Hold", "Run"})  [unwired: 2 in]
        n67 = local write "Mode 1"(w180) -> ()
        n68 = local write "Mode"(w180) -> ()
        n69 = case shown="\"Hold\"" w175 {
          tunnel: [w183 TRUE ("On/Off") TRUE ("On/Off") TRUE ("On/Off")] -> w176
          tunnel: [w183 FALSE ("On/Off") FALSE ("On/Off") TRUE ("On/Off")] -> w173
          frame "Off", Default {
            w183 = FALSE ("On/Off")
          }
          frame "Stby" {
          }
          frame "Hold" {
          }
          frame "Run" {
          }
        }
        n70 = local write "Mode Select"(w175) -> ()
        n71 = call "Call Power On-Off.vi"("error in"=w179, "Warmup if ON"=w173, "VISA resource name"=w177, "On/Off"=w176) -> ("error out"=w178:errorcluster)  [unwired: 1 in, 1 out]
      }
      event Value Change {
        n72 = event-data() -> ("OldVal"=w199:T10, "NewVal"=w198:T10)  [unwired: 1 in, 3 out]
        n73 = Not Equal?(x=w199, y=w198) -> (x != y?=w197:T10)
        n74 = call "4 Way Sub.vi"("OldVal"=w197) -> ("Mode Select"=w192:enum8{"Off", "Stby", "Hold", "Run"})  [unwired: 2 in]
        n75 = local write "Mode Select"(w192) -> ()
        n76 = local write "Mode 1"(w197) -> ()
        n77 = local write "Mode"(w197) -> ()
        n78 = case shown="\"Hold\"" w192 {
          tunnel: [w200 TRUE ("On/Off") TRUE ("On/Off") TRUE ("On/Off")] -> w190
          tunnel: [w200 FALSE ("On/Off") FALSE ("On/Off") TRUE ("On/Off")] -> w191
          frame "Off", Default {
            w200 = FALSE ("On/Off")
          }
          frame "Stby" {
          }
          frame "Hold" {
          }
          frame "Run" {
          }
        }
        n79 = call "Call Power On-Off.vi"("error in"=w196, "Warmup if ON"=w191, "VISA resource name"=w194, "On/Off"=w190) -> ("error out"=w195:errorcluster)  [unwired: 1 in, 1 out]
      }
      event "Confirm Now": Value Change {
        n80 = event-data() -> ()  [unwired: 1 in, 5 out]
        n81 = local write "ALT SET 2"("ALT SET") -> ()
        n82 = call "Alt 2 Num.vi"("Alt Ctl"="ALT SET") -> ("Alt"=w208:i32)  [unwired: 2 in]
      }
      event "Confirm Now 2": Value Change {
        n83 = event-data() -> ()  [unwired: 1 in, 5 out]
        n84 = local write "ALT SET"("ALT SET 2") -> ()
        n85 = call "Alt 2 Num.vi"("Alt Ctl"="ALT SET 2") -> ("Alt"=w210:i32)  [unwired: 2 in]
      }
      event Value Change {
        n86 = event-data() -> ()  [unwired: 1 in, 5 out]
      }
    }
    "CURRENT ALT SET 2" <- w163
    "CURRENT ALT SET" <- w163
    n87 = local write "Set Point Alt"(w163) -> ()
  }
  n88 = node-c288(w34) -> ()  [unwired: 1 out]
  n89 = call "Call Power On-Off.vi"("error in"=w24, "Warmup if ON"=w1, "VISA resource name"=w20, "On/Off"=w1) -> ("error out"=w4:errorcluster, "VISA resource name out"=w5:refnum<visa-resource-name>)  [unwired: 1 in]
  n90 = VISA Clear(VISA resource name=w5, error in (no error)=w4) -> (error out=w3:errorcluster)  [unwired: 1 out]
  n91 = Merge Errors(w3, w26) -> (w25:errorcluster)
  n92 = local write "error out"(w25) -> ()
